vi "test imaq create string and string to array dlls.vi"() -> ()   [LabVIEW 2020]
uses:
  GEECS-Plugins/tcp client/CreateExampleIMAQString.dll
panel:
  out "Data String":string
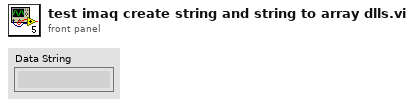
[diagram p1: front panel]
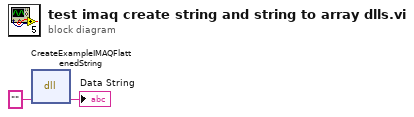
[diagram p0: block diagram]
diagram:
  n1 = dll-call lib="C:/GEECS/Developers Version/source/GEECS-Plugins/tcp client/CreateExampleIMAQString.dll" fn="CreateExampleIMAQFlattenedString"("Data String"="") -> ("Data String"=→"Data String":string)  [unwired: 4 in, 2 out]
